vi "Create Thread Section.vi"(7 "GUID (Default Section)":string="03D3BB89-1485-13A6-56005DE6430FF8B7", 8 "error in (no error)":errorcluster, 10 "Thread Configurations":refnum<class "Thread Configuration.lvclass">[](array[class]), 11 "Item Ref in":T1 format="%.0x") -> (0 "error out":errorcluster, 2 "Thread Section refs":T1[](array[typedef]) format="%.0x", 3 "Item Ref out":T1 format="%.0x")   [LabVIEW 2019, in "DSF System Explorer.lvlib"]
uses:
  DSF System Explorer.lvlib
  <vilib>/NI VeriStand/Custom Device API/Custom Device API.lvlib
  <vilib>/NI VeriStand/Custom Device API/Custom Device Item Ref.ctl
  DSF Core.lvlibp/Classes/Configuration/Core/Thread/Thread Configuration.lvclass
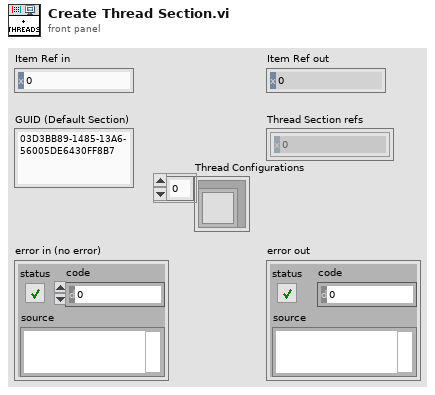
[diagram p1: front panel]
types:
  T1 = typedef "Custom Device API.lvlib/Custom Device Item Ref.ctl" = u64
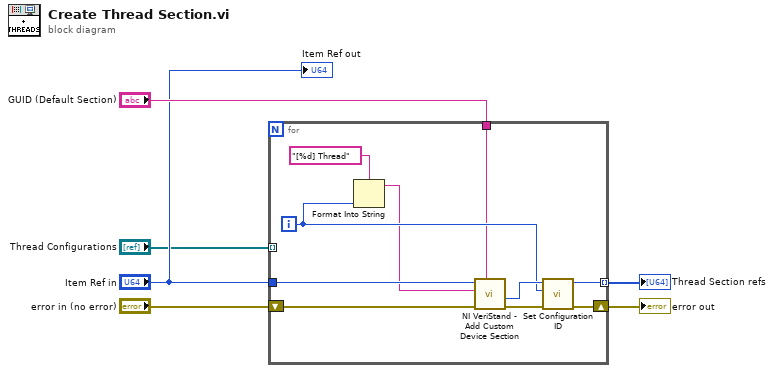
[diagram p0: block diagram]
diagram:
  n1 = for {
    tunnel: "Item Ref in" -> [w15]
    shift-right: [w11] -> w6
    shift-left: "error in (no error)" -> [w10]
    tunnel: [w12] -> w5 mode=indexing
    tunnel: "GUID (Default Section)" -> [w8]
    tunnel: "Thread Configurations" -> [_] mode=indexing
    i -> [w9]
    n2 = Format Into String(format string="[%d] Thread", w9) -> (resulting string=w7:string)  [unwired: 2 in, 1 out]
    n3 = call <vilib>:"NI VeriStand - Add Custom Device Section.vi"("GUID (Default Section)"=w8, "error in (no error)"=w10, "Section Name"=w7, "Parent Ref in"=w15) -> ("error out"=w13:errorcluster, "Section Ptr"=w14:T1)  [unwired: 4 in, 2 out]
    n4 = call "Set Configuration ID.vi"("error in (no error)"=w13, "Configuration ID"=w9, "Item Ref in"=w14) -> ("error out"=w11:errorcluster, "Item Ref out"=w12:T1)  [unwired: 7 in]
  }
  "error out" <- w6
  "Thread Section refs" <- w5
  "Item Ref out" <- "Item Ref in"
